vi "CSM Execute - Go to State.vi"(6 "Mouse Position":T1, 8 "User VI Ref":refnum<vi>, 9 "Menu Item Tag Suffix":string, 10 "Remaining Items":refnum<vi>[](array[refnum]), 11 "Affected Items":T2) -> (0 "Fail transaction?":bool)   [LabVIEW 2017]
doc: "This VI is part of a plug-in for modifying the LabVIEW shortcut menus. This is the execute VI which is called when the shortcut menu is chosen by the user. It performs the action of the selected menu item."
uses:
  CSM Execute - Shortcut Menu Plug-In.ctl
  <vilib>/Utility/miscctls.llb/LVPositionTypeDef.ctl
  _csmHelper/API with lvcsm Support/CSM-Helper API with lvcsm Support.lvlib
panel:
  # "All controls on this panel except \"Affected Items\" have been locked to prevent accidental edits. Changing the control names or types, other than the elements of the \"Affected Items\" cluster will make the VI unusable as a menu plugin.\n\nSee Context Help for each control for details about its use."
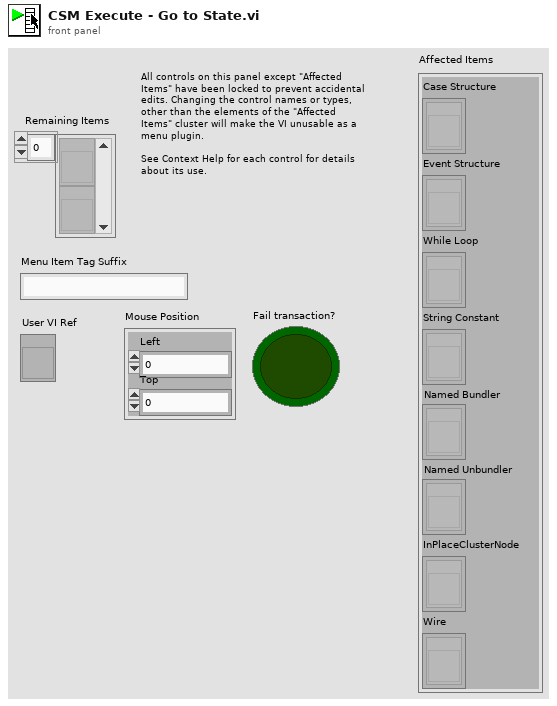
[diagram p1: front panel]
types:
  T1 = typedef "LVPositionTypeDef.ctl" = cluster{"Left":i32, "Top":i32}
  T2 = typedef "CSM Execute - Shortcut Menu Plug-In.ctl" = cluster{"Case Structure":refnum<vi>[], "Event Structure":refnum<vi>[], "While Loop":refnum<vi>[], "String Constant":refnum<vi>[], "Named Bundler":refnum<vi>[], "Named Unbundler":refnum<vi>[], "InPlaceClusterNode":refnum<vi>[], "Wire":refnum<vi>[]}
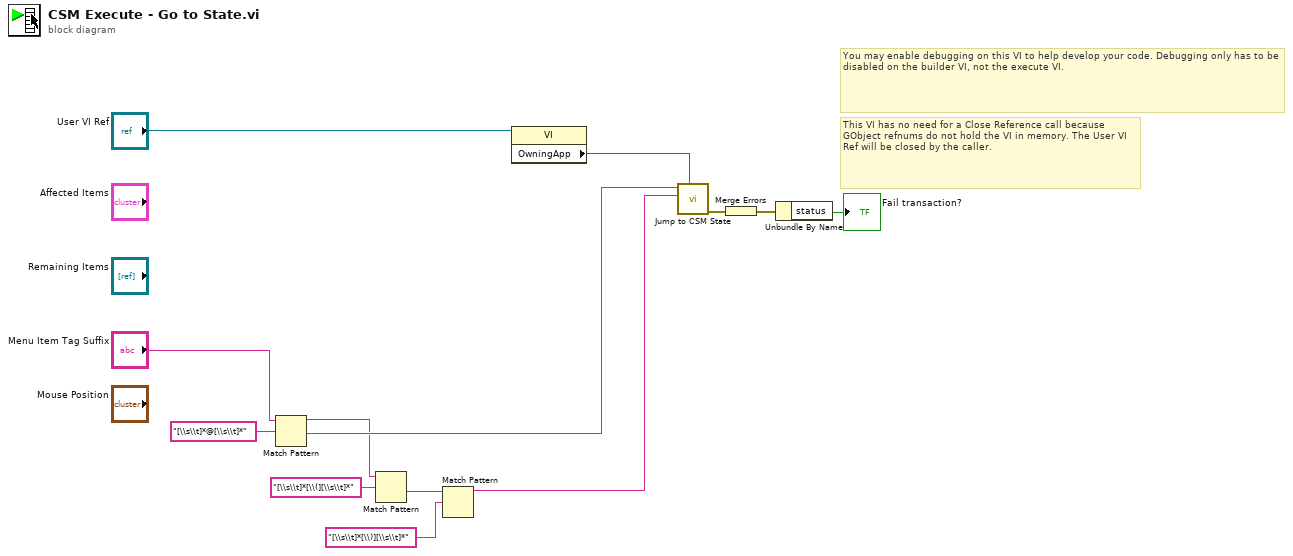
[diagram p0: block diagram]
diagram:
  # "You may enable debugging on this VI to help develop your code. Debugging only has to be disabled on the builder VI, not the execute VI."
  # "This VI has no need for a Close Reference call because GObject refnums do not hold the VI in memory. The User VI Ref will be closed by the caller."
  n1 = Match Pattern(string="Menu Item Tag Suffix", regular expression="[\\s\\t]*@[\\s\\t]*") -> (before substring=w2:string, after substring=w3:string)  [unwired: 1 in, 2 out]
  n2 = Match Pattern(string=w2, regular expression="[\\s\\t]*[\\(][\\s\\t]*") -> (after substring=w6:string)  [unwired: 1 in, 3 out]
  n3 = Match Pattern(string=w6, regular expression="[\\s\\t]*[\\)][\\s\\t]*") -> (before substring=w1:string)  [unwired: 1 in, 3 out]
  n4 = property class="VI"(reference="User VI Ref") -> ("OwningApp"=w9:refnum<vi>)  [unwired: 1 in, 2 out]
  n5 = call "Jump to CSM State.vi"("Application Reference (Local)"=w9, "State"=w1, "Name"=w3) -> ("error out"=w11:errorcluster)  [unwired: 8 in]
  n6 = Merge Errors(w11) -> (w12:errorcluster)
  n7 = Unbundle By Name(w12) -> ("status"=→"Fail transaction?":bool)
